vi "S2C_OM8257_Poly_ACW.vi"(8 "Error In":errorcluster, 10 "ACW":T1={"Voltage (V)"=1240, "High Limit Total (mA)"=10.0, "Low Limit Total (mA)"=0.0, "Ramp Up Time (s)"=0.1, "Dwell Time (s)"=1.0, "Arc Sense"=5, "Arc Detect"=FALSE, "High Limit Real (mA)"=10.0, "Low Limit Real (mA)"=0.0, "Ramp Down Time (s)"=0.0, "Continuity"=FALSE, "Offset (mA)"=0.0, "Auto Offset"=FALSE, "DUT Output"=FALSE, "Frequency (Hz)"=60, "Scanner?"=FALSE, "Step Selection"=1, "Add Step"=FALSE, "Scan1"=1, "Scan2"=1, "Scan3"=1, "Scan4"=1, "Scan5"=1, "Scan6"=1, "Scan7"=1, "Scan8"=1, "Scan9"=1, "Scan10"=1, "Scan11"=1, "Scan12"=1, "Scan13"=1, "Scan14"=1, "Scan15"=1, "Scan16"=1} {"Scan16" min=0 max=2 step=1; "Scan15" min=0 max=2 step=1; "Scan14" min=0 max=2 step=1; "Scan13" min=0 max=2 step=1; "Scan12" min=0 max=2 step=1; "Scan11" min=0 max=2 step=1; "Scan10" min=0 max=2 step=1; "Scan9" min=0 max=2 step=1; "Scan8" min=0 max=2 step=1; "Scan7" min=0 max=2 step=1; "Scan6" min=0 max=2 step=1; "Scan5" min=0 max=2 step=1; "Scan4" min=0 max=2 step=1; "Scan3" min=0 max=2 step=1; "Scan2" min=0 max=2 step=1; "Scan1" min=0 max=2 step=1}, 11 "Settings":T2={"Driver"="Omnia8257", "Command"="CfgStep ACW", "Return"="ErrorStatus", "Parameters"="", "Timeout"=10.0}) -> (0 "Error Out":errorcluster, 3 "Response":string)   [LabVIEW 2015]
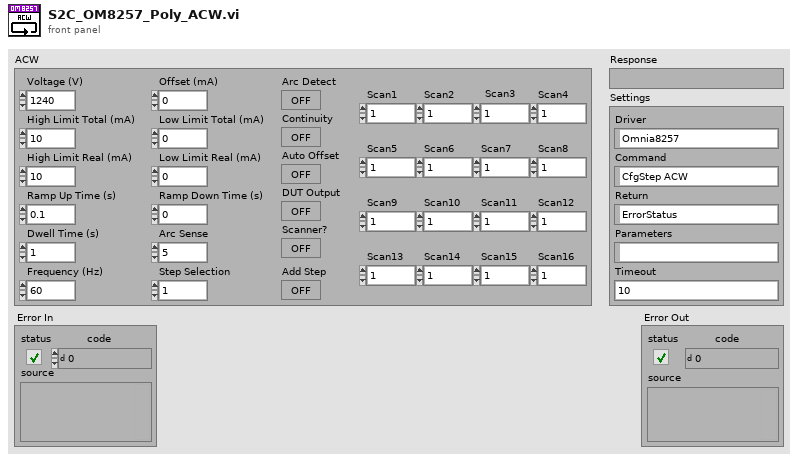
[diagram p1: front panel]
types:
  T1 = cluster{"Voltage (V)":u16, "High Limit Total (mA)":dbl, "Low Limit Total (mA)":dbl, "Ramp Up Time (s)":dbl, "Dwell Time (s)":dbl, "Arc Sense":u8, "Arc Detect":bool, "High Limit Real (mA)":dbl, "Low Limit Real (mA)":dbl, "Ramp Down Time (s)":dbl, "Continuity":bool, "Offset (mA)":dbl, "Auto Offset":bool, "DUT Output":bool, "Frequency (Hz)":u16, "Scanner?":bool, "Step Selection":i32, "Add Step":bool, "Scan1":i32, "Scan2":i32, "Scan3":i32, "Scan4":i32, "Scan5":i32, "Scan6":i32, "Scan7":i32, "Scan8":i32, "Scan9":i32, "Scan10":i32, "Scan11":i32, "Scan12":i32, "Scan13":i32, "Scan14":i32, "Scan15":i32, "Scan16":i32}
  T2 = cluster{"Driver":string, "Command":string, "Return":string, "Parameters":string, "Timeout":dbl}
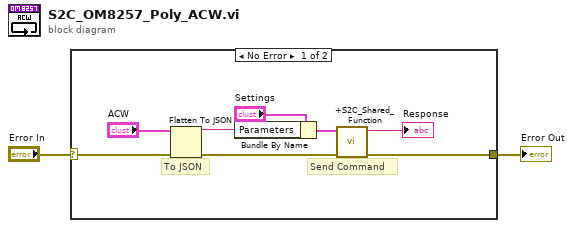
[diagram p0: block diagram]
diagram:
  n1 = case shown="No Error" "Error In" {
    selector: "Error In" -> [w6 w11]
    tunnel: [w5 w11] -> w1
    frame No Error {
      # "To JSON"
      # "Send Command"
      n2 = Flatten To JSON(anything="ACW", error in (no error)=w6) -> (JSON string=w7:string, 11:w9:errorcluster)  [unwired: 1 in]
      n3 = Bundle By Name(cluster="Settings", "Parameters"=w7) -> (w10:T2)
      n4 = call "+S2C_Shared_Function.vi"("Error In"=w9, "Settings"=w10) -> ("Error Out"=w5:errorcluster, "Response"=→"Response":string)  [unwired: 8 in]
    }
    frame Error {
    }
  }
  "Error Out" <- w1
